vi "lib Delete Files and Folders.vi"(8 "error in (no error)":errorcluster, 10 "Include Sub Folders?":bool, 11 "Path to Folder":path) -> (0 "error out":errorcluster)   [LabVIEW 2015]
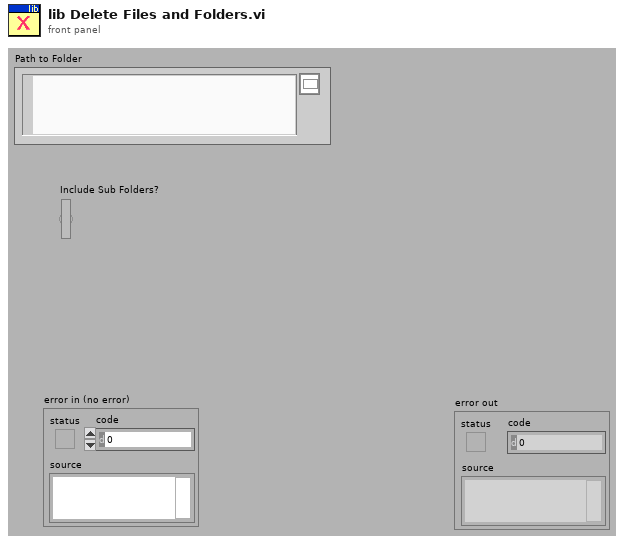
[diagram p1: front panel]
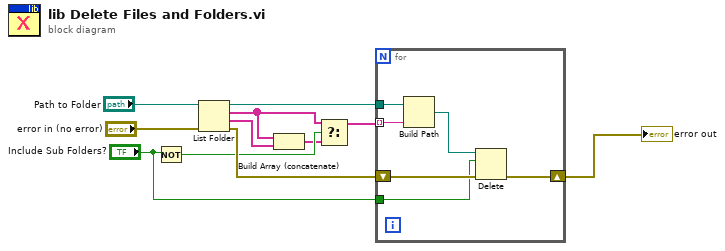
[diagram p0: block diagram]
diagram:
  n1 = Not(x="Include Sub Folders?") -> (.not. x?=w4:bool)
  n2 = List Folder(path="Path to Folder", error in="error in (no error)") -> (path out=w11:path, filenames=w5:string[], folder names=w6:string[], error out=w9:errorcluster)  [unwired: 2 in]
  n3 = Build Array (concatenate)(w5, w6) -> (w3:string[])
  n4 = Select(t=w5, s=w4, f=w3) -> (s? t:f=w2:string[])
  n5 = for {
    tunnel: w11 -> [w17]
    tunnel: w2 -> [w13] mode=indexing
    shift-right: [w14] -> w8
    shift-left: w9 -> [w15]
    tunnel: "Include Sub Folders?" -> [w12]
    n6 = Build Path(base path=w17, name or relative path=w13) -> (appended path=w16:path)
    n7 = Delete(path (use dialog)=w16, entire hierarchy (F)=w12, error in=w15) -> (error out=w14:errorcluster)  [unwired: 2 in, 2 out]
  }
  "error out" <- w8
